vi "SPD.Dequeue State.vi"(8 "Error In":errorcluster, 11 "SPD.Stand Ctrl in":T2 {"spdDeviceSession"."hidSPD.Sturtup Values"."HV_bias" format="%#_6p, V"; "spdDeviceSession"."hidSPD.Sturtup Values"."TSet" format="%#_6p, DegC"; "spdDeviceSession"."hidSPD.Controller"."HV_bias" format="%#_6p, V"; "spdDeviceSession"."hidSPD.Controller"."TSet" format="%#_6p, DegC"}) -> (0 "Error Out":errorcluster, 2 "SPD.state":T1, 3 "SPD.Stand Ctrl out":T2 {"spdDeviceSession"."hidSPD.Sturtup Values"."HV_bias" format="%#_6p, V"; "spdDeviceSession"."hidSPD.Sturtup Values"."TSet" format="%#_6p, DegC"; "spdDeviceSession"."hidSPD.Controller"."HV_bias" format="%#_6p, V"; "spdDeviceSession"."hidSPD.Controller"."TSet" format="%#_6p, DegC"})   [LabVIEW 2018]
uses:
  typedefs/SPD.Stand Ctrl.ctl
  Instruments/SPD HID Interface/hidSPDLibForLabView/LibVIs/hidSPD Controls/hidSPD Device Session.ctl
  Instruments/SPD HID Interface/hidSPDLibForLabView/LibVIs/hidSPD Controls/hidSPD Controller.ctl
  Instruments/SPD HID Interface/hidSPDLibForLabView/LibVIs/hidSPD Controls/hidSPD SPD Type.ctl
  Instruments/KC705 DevBoard/typedefs/DevB.Session.ctl
  Instruments/KeySight 53230A/typedefs/FreqC.Session.ctl
  Instruments/KeySight 8164B/KeySight 8164B LAN InstrLib/typedefs/KeySight 8164B control.ctl
  Instruments/LeCroy SDA830/typedefs/LeCroy.Session.ctl
  typedefs/SPD.Events.ctl
  ConfigFile/SPD.Config File ctrl.ctl
  <vilib>/Utility/config.llb/Config Data RefNum.ctl
  typedefs/SPD.Meas Result.ctl
  typedefs/SPD.Queues.ctl
  typedefs/SPD.Stand state.ctl
  Instruments/KeySight 8164B/KeySight 8164B LAN InstrLib.lvlib
  <vilib>/Utility/config.llb/NI_LVConfig.lvlib
  Instruments/SPD HID Interface/hidSPDLibForLabView/hidSPDLibForLabView.lvlib
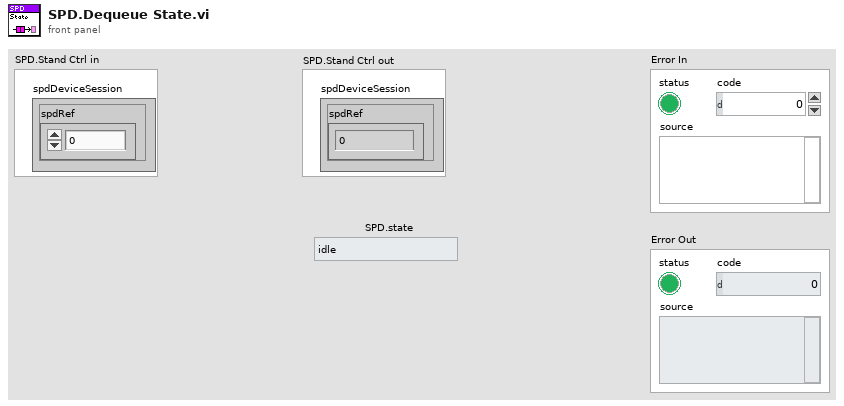
[diagram p1: front panel]
types:
  T1 = typedef "SPD.Stand state.ctl" = enum16{"idle", "HW.Conect", "HW.FreqC selftest", "HW.8164B selftest", "HW.Scope selftest", "HW.KC705 selftest", "HW.Laser test", "HW.Power source test", "SPD.connect", "SPD.set type", "SPD.write", "SPD.read", "SPD.tests", "Meas.Grid update", "Meas", "App.Handle Error", "App.Stop"}
  T2 = typedef "SPD.Stand Ctrl.ctl" = cluster{"spdDeviceSession":T3, "DevBSession":T6, "FreqCSession":T7, "8164BSession":T8, "LeCroySession":T9, "Events":T10, "configFile":T11, "SPD.Result":T13, "SPD.Queues":T14, "Console":refnum<vi>}
  T3 = typedef "hidSPDLibForLabView.lvlib/hidSPD Device Session.ctl" = cluster{"spdRef":u64, "connected":bool, "spdName":string, "hidSPD.Controller":T4, "hidSPD.Sturtup Values":T4, "SPD Type":T5}
  T4 = typedef "hidSPDLibForLabView.lvlib/hidSPD Controller.ctl" = cluster{"TSet":sgl, "HV_bias":sgl, "DDS_stb_code":u16}
  T5 = typedef "hidSPDLibForLabView.lvlib/hidSPD SPD Type.ctl" = enum16{"Free Run", "Strobe"}
  T6 = typedef "DevB.Session.ctl" = cluster{"DevBRef":refnum<visa-resource-name>, "connected":bool}
  T7 = typedef "FreqC.Session.ctl" = cluster{"FreqCRef":refnum<visa-resource-name>, "timeout":dbl, "Gate":dbl, "connected":bool}
  T8 = typedef "KeySight 8164B LAN InstrLib.lvlib/KeySight 8164B control.ctl" = cluster{"Connection ID":refnum<k5>, "Connected":bool, "Info":string, "Slots Info":string[]}
  T9 = typedef "LeCroy.Session.ctl" = cluster{"LeCroySession":refnum<visa-resource-name>, "connected":bool}
  T10 = typedef "SPD.Events.ctl" = cluster{"DCRTest":refnum<user-event>, "Stop":refnum<user-event>}
  T11 = typedef "SPD.Config File ctrl.ctl" = cluster{"configFile ref":T12, "configFile path":path, "equipmentFile ref":T12}
  T12 = typedef "NI_LVConfig.lvlib/Config Data RefNum.ctl" = refnum<k1>
  T13 = typedef "SPD.Meas Result.ctl" = cluster{"HV_Bias":dbl[][][], "Stb_code":dbl[], "Temprature":dbl[], "Data":dbl[][][][], "DateTime":string}
  T14 = typedef "SPD.Queues.ctl" = cluster{"state queue":refnum<queue>}
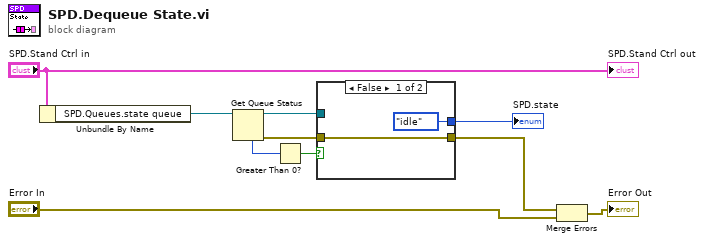
[diagram p0: block diagram]
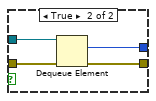
[diagram p2: hidden frame]
diagram:
  n1 = Unbundle By Name("SPD.Stand Ctrl in") -> ("SPD.Queues.state queue"=w9:refnum<queue>)
  n2 = Get Queue Status(queue=w9) -> (queue out=w6:refnum<queue>, error out=w5:errorcluster, # elements in queue=w8:i32)  [unwired: 2 in, 5 out]
  n3 = Greater Than 0?(x=w8) -> (x > 0?=w7:bool)
  n4 = case shown="False" w7 {
    tunnel: w6 -> [_ w16]
    tunnel: w5 -> [w11 w15]
    tunnel: [w11 w14] -> w4
    tunnel: [SPD.Stand_state."idle" ("SPD.stand state") w13] -> w3
    frame False {
    }
    frame True {
      n5 = Dequeue Element(queue=w16, error in (no error)=w15) -> (element=w13:T1, error out=w14:errorcluster)  [unwired: 1 in, 2 out]
    }
  }
  "SPD.state" <- w3
  n6 = Merge Errors(w4, "Error In") -> (→"Error Out":errorcluster)
  "SPD.Stand Ctrl out" <- "SPD.Stand Ctrl in"
